vi "List Project Files with Specified Pattern_lvcicd.vi"(8 "error in (no error)":errorcluster, 10 "pattern":string="_build.*.lvproj", 11 "Path":path=path "D:/Workspace") -> (0 "error out":errorcluster, 1 "No Index Project":path[](array[path]), 3 "All Files in Dir":path[](array[path]))   [LabVIEW 2014, in "_lvcicd_support_2014.lvlib"]
uses:
  <userlib>/_OpenG.lib/array/array.llb/Sort 1D Array (I32)__ogtk.vi
  <userlib>/_OpenG.lib/array/array.llb/Index 1D Array Elements (Path)__ogtk.vi
  _lvcicd_support_2014.lvlib
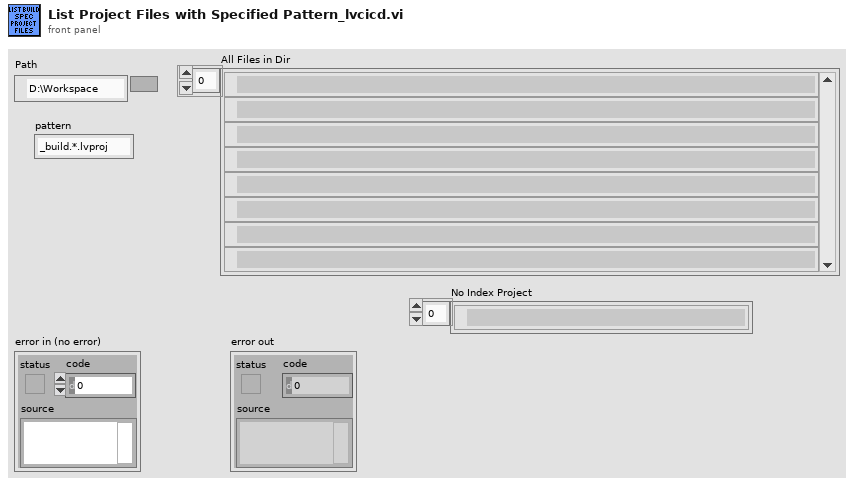
[diagram p1: front panel]
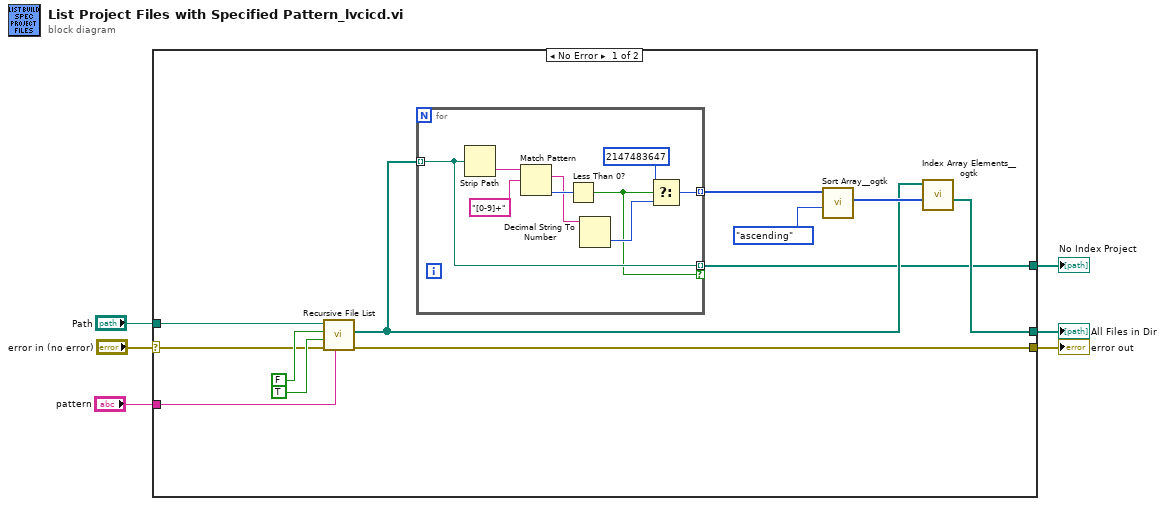
[diagram p0: block diagram]
diagram:
  n1 = case shown="No Error" "error in (no error)" {
    selector: "error in (no error)" -> [w15 w28]
    tunnel: "Path" -> [w18 _]
    tunnel: [w9 _] -> w5
    tunnel: [w14 w28] -> w3
    tunnel: [w8 _] -> w2
    tunnel: "pattern" -> [w7 _]
    frame No Error {
      n2 = call <vilib>:"Recursive File List.vi"("pattern"=w7, "error in (no error)"=w15, "Continue Recursing on Error? (F)"=TRUE, "Treat LLBs as Folders?"=FALSE, "Folder Path"=w18) -> ("error out"=w14:errorcluster, "All Files in Dir"=w10:path[])  [unwired: 2 in, 3 out]
      n3 = for {
        tunnel: w10 -> [w20] mode=indexing
        tunnel: [w21] -> w13 mode=indexing
        tunnel: [w20] -> w8 mode=indexing if=w19
        n4 = Strip Path(path=w20) -> (name=w27:string)  [unwired: 1 out]
        n5 = Match Pattern(string=w27, regular expression="[0-9]+") -> (match substring=w23:string, offset past match=w25:i32)  [unwired: 1 in, 2 out]
        n6 = Less Than 0?(x=w25) -> (x < 0?=w19:bool)
        n7 = Decimal String To Number(string=w23) -> (number=w22:i32)  [unwired: 2 in, 1 out]
        n8 = Select(t=2147483647, s=w19, f=w22) -> (s? t:f=w21:i32)
      }
      n9 = call-poly <userlib>:"Sort Array__ogtk.vi"("Order"=enum16{"ascending", "descending"}."ascending", "Array in"=w13) -> ("Sorted Pointers"=w11:i32[])  [unwired: 8 in, 1 out]
      n10 = call-poly <userlib>:"Index Array Elements__ogtk.vi"("indices"=w11, "array"=w10) -> ("elements"=w9:path[])  [unwired: 9 in]
    }
    frame Error {
    }
  }
  "All Files in Dir" <- w5
  "error out" <- w3
  "No Index Project" <- w2
